vi "Alazartech_Data_fetching.vi"(0 "Rec/Buf":u32=128, 3 "RecordLength":u32=4096, 4 "Trig. Delay (us)":sgl=6.5, 5 "Triger Source":T1(ring)=enum."External", 7 "9350_Range":u32(ring)=6 items=["40mV", "100mV", "200mV", "400mV", "1 V", "2 V", "4 V"], 9 "Device":i32) -> (1 "Error":bool, 2 "DeviceOut":i32)   [LabVIEW 2009]
uses:
  C:/AlazarTech/ATS-VI/5.8.3/ATS_ctl/ATS_Async_Ctrl.ctl
panel:
  in  "Level":u32=181
  out "PLL Locked":bool
  in  "Display":bool
  out "Waveform Graph":u16[](graph)
  out "Valid":bool
  out "Get Data Status":string
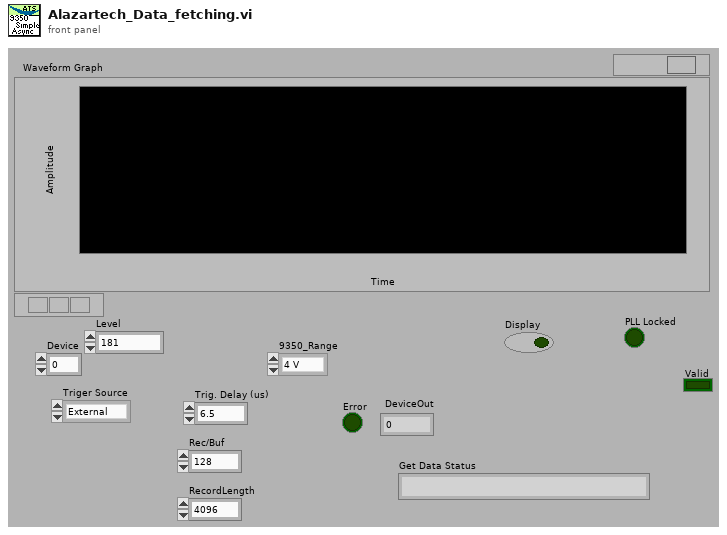
[diagram p1: front panel]
types:
  T1 = enum32{"Chan_A", "Chan_B", "External", "Disable"}
  T2 = typedef "ATS_Async_Ctrl.ctl" = enum16{"SetupDMA", "StartCapture", "Get", "Get_Stream", "Abort", "Stop"}
  T3 = typedef "ATS_Async_Status.ctl" = cluster{"Start DMA":bool, "StartCapture":bool, "Valid":bool, "Completed":bool, "InProgress":bool, "Timeout":bool, "Overflow":bool, "Error":bool}
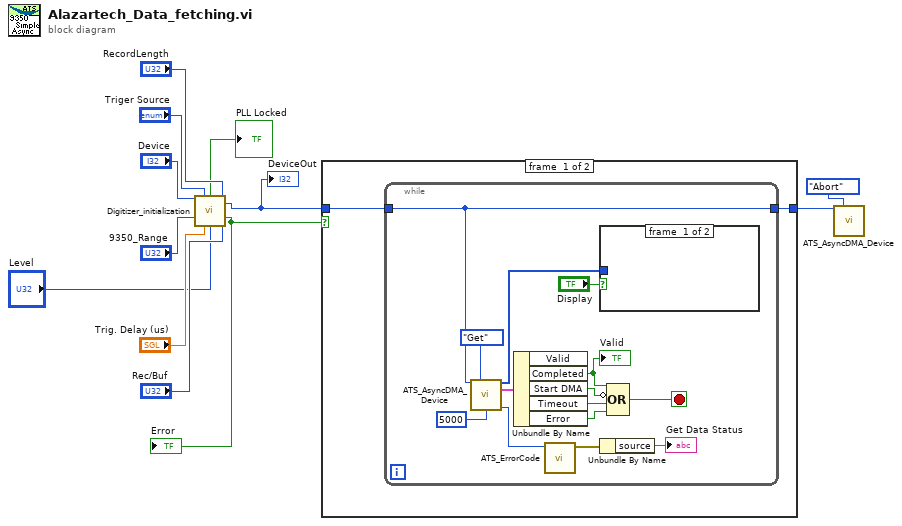
[diagram p0: block diagram]
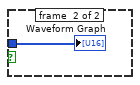
[diagram p2: hidden frame]
diagram:
  n1 = call "Digitizer_initialization.vi"("Device"="Device", "Triger Source"="Triger Source", "RecordLength"="RecordLength", "9350_Range"="9350_Range", "Trig. Delay (us)"="Trig. Delay (us)", "Level"="Level", "Rec/Buf"="Rec/Buf") -> ("PLL Locked"=→"PLL Locked":bool, "DeviceOut"=w3:i32, "Error"=w4:bool)  [unwired: 6 in]
  "DeviceOut" <- w3
  "Error" <- w4
  n2 = case shown="False" w4 {
    tunnel: w3 -> [w14 w30]
    tunnel: [w13 w30] -> w11
    frame #0 {
      n3 = while {
        tunnel: w14 -> [w22]
        tunnel: [w22] -> w13
        stop <- w18 stop-if-true
        n4 = call "ATS_AsyncDMA_Device.vi"("DeviceIn"=w22, "ATS_Async_Ctrl"=ATS_Async_Ctrl."Get", "WaitTimeOut (ms)"=u32 5000) -> ("Buffer"=w23:u16[], "Async_Status"=w25:T3, "Return Code"=w19:u32)  [unwired: 5 in, 5 out]
        n5 = Unbundle By Name(w25) -> ("Completed"=w15:bool, "Start DMA"=w28:bool, "Timeout"=w27:bool, "Error"=w26:bool)  [unwired: 1 out]
        "Valid" <- w15
        n6 = call "ATS_ErrorCode.vi"("ErrorCode"=w19) -> ("error out"=w21:errorcluster)  [unwired: 1 in, 5 out]
        n7 = case shown="True" "Display" {
          tunnel: w23 -> [_ w29]
          frame #0 {
          }
          frame #1 {
            "Waveform Graph" <- w29
          }
        }
        n8 = Unbundle By Name(w21) -> ("source"=→"Get Data Status":string)
        n9 = Compound Arithmetic op=OR(w15, invert w28, w27, w26) -> (w18:bool)
      }
    }
    frame #1 {
    }
  }
  n10 = call "ATS_AsyncDMA_Device.vi"("DeviceIn"=w11, "ATS_Async_Ctrl"=ATS_Async_Ctrl."Abort" ("ATS_DMA_Ctrl")) -> ()  [unwired: 6 in, 8 out]
